vi "sinenoisebd.vi"() -> ()   [LabVIEW 2023]
uses:
  <vilib>/Analysis/2dsp.llb/Real FFT.vi
  <vilib>/Analysis/3filter.llb/Butterworth Filter (DBL).vi
  <vilib>/measure/NI_MABase.lvlib
  <vilib>/Analysis/NI_AALBase.lvlib
  <vilib>/Analysis/NI_AALPro.lvlib
panel:
  out "Waveform Graph 4":dbl[](graph)
  out "Waveform Graph 3":dynamicdata(graph)
  out "Waveform Graph 2":dbl[](graph)
  in  "stop":bool
  out "Waveform Graph":waveform(dbl)(graph)
  in  "amplitude":dbl(knob)=1.0 scale=0.0..10.0
  in  "frequency":dbl(knob)=10.0 scale=0.0..10.0
  in  "offset":dbl(slide) scale=0.0..10.0
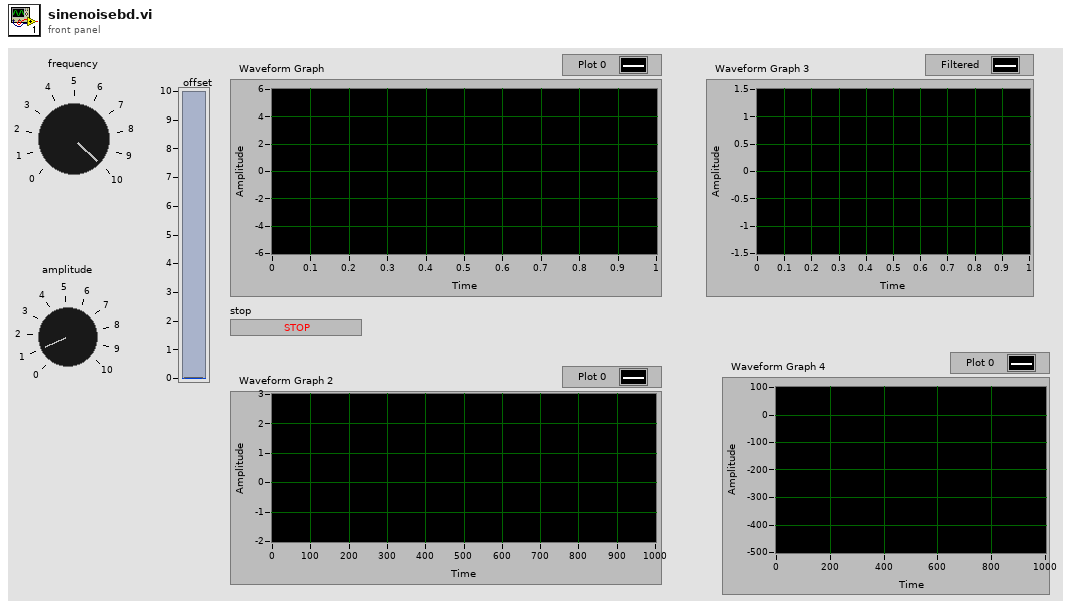
[diagram p1: front panel]
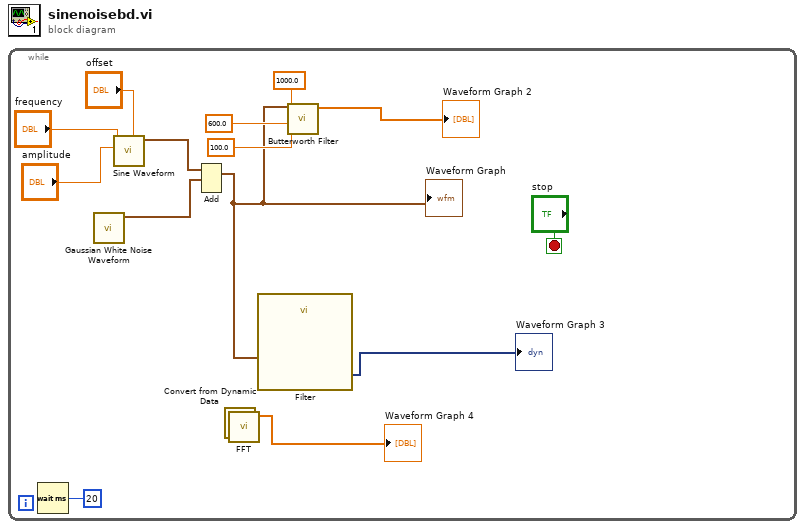
[diagram p0: block diagram]
diagram:
  n1 = while {
    stop <- "stop" stop-if-true
    n2 = Wait (ms)(milliseconds to wait=u32 20) -> ()  [unwired: 1 out]
    n3 = call <vilib>:"Gaussian White Noise Waveform.vi"() -> ("signal out"=w10:waveform(dbl))  [unwired: 10 in, 1 out]
    n4 = call <vilib>:"Sine Waveform.vi"("offset"="offset", "amplitude"="amplitude", "frequency"="frequency") -> ("signal out"=w9:waveform(dbl))  [unwired: 7 in, 1 out]
    n5 = Add(1:w10, 2:w9) -> (0:w3:waveform(dbl))  [unwired: 1 in, 1 out]
    "Waveform Graph" <- w3
    n6 = call "Convert from Dynamic Data"() -> ("Array"=w2:dbl[])  [unwired: 4 in]
    n7 = call-poly <vilib>:"FFT.vi"("X"=w2) -> ("FFT {X}"=→"Waveform Graph 4":cdb[])  [unwired: 9 in, 1 out]
    n8 = call "Filter"("Signal"=w3) -> ("Filtered Signal"=→"Waveform Graph 3":dynamicdata)  [unwired: 9 in, 1 out]
    n9 = call-poly <vilib>:"Butterworth Filter.vi"("low cutoff freq: fl"=100.0, "high cutoff freq: fh"=600.0, "sampling freq: fs"=1000.0, "X"=w3) -> ("Filtered X"=→"Waveform Graph 2":dbl[])  [unwired: 4 in, 1 out]
  }
